vi "Panel.vi"(11 "SerialConfigPanel in":refnum<class "SerialConfigPanel.lvclass">) -> ()   [LabVIEW 2020, in "LV-Term.lvlib" / "SerialConfigPanel.lvclass"]
uses:
  SerialConfigPanel.lvclass
  SerialConfigPanel.lvclass/SerialConfigPanel.ctl
  <vilib>/IlluminatedG/IG OOPanel/OOPanel/Panel/Basic UI State.ctl
  <vilib>/IlluminatedG/IG OOPanel/OOPanel/Panel/Panel.lvclass
  <vilib>/IlluminatedG/IG OOPanel/OOPanel/OOPanel.lvlib
  C:/Program Files (x86)/National Instruments/LabVIEW 2020/vi.lib/IlluminatedG/IG OOPanel/OOPanel/Panel/Panel.lvclass
  C:/dev/illuminated-g/lv-terminal-app/LV-Term/SerialConfigPanel/SerialConfigPanel.lvclass
  C:/dev/illuminated-g/lv-terminal-app/LV-Term/ConfigPanel/ConfigPanel.lvclass
  <vilib>/IlluminatedG/IG Serial Stream/Stream-Serial/Serial Client/Stop Bits.ctl
  <vilib>/IlluminatedG/IG Serial Stream/Stream-Serial/Serial Client/Serial Client.lvclass
  <vilib>/IlluminatedG/IG Serial Stream/Stream-Serial/Serial Client/Flow Control.ctl
  <vilib>/IlluminatedG/IG Serial Stream/Stream-Serial/Serial Client/Parity.ctl
panel:
  in  "Port":refnum<visa-resource-name>
  in  "Timeout ms":i32=10000
  in  "Parity":T1
  in  "Flow Control":T2 items=["None", "XON/XOFF", "RTS/CTS", "XON/XOFF & RTS/CTS", "DTR/DSR", "XON/XOFF & DTR/DSR"]
  in  "Stop Bits":T3=10 items=["1.0"=10, "1.5"=15, "2.0"=20]
  in  "Data Bits":u8=8
  in  "Baud":u32=115200
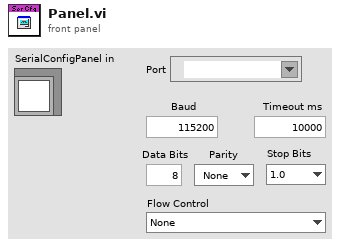
[diagram p1: front panel]
types:
  T1 = typedef "Stream-Serial.lvlib/Serial Client.lvclass/Parity.ctl" = enum16{"None", "Odd", "Even", "Mark", "Space"}
  T2 = typedef "Stream-Serial.lvlib/Serial Client.lvclass/Flow Control.ctl" = u16
  T3 = typedef "Stream-Serial.lvlib/Serial Client.lvclass/Stop Bits.ctl" = u16
  T4 = typedef "OOPanel.lvlib/Panel.lvclass/Basic UI State.ctl" = enum16{"Init", "Run", "Close"}
  T5 = typedef "OOPanel.lvlib/Panel.lvclass/Panel Events.ctl" = cluster{"Visbility":refnum<user-event>, "Close":refnum<user-event>}
  T6 = typedef "LV-Term.lvlib/SerialConfigPanel.lvclass/Ref Data.ctl" = cluster{"Port":refnum<visa-resource-name>, "Config":T7}
  T7 = typedef "Stream-Serial.lvlib/Serial Client.lvclass/Port Config.ctl" = cluster{"Baud (115200)":u32, "Data Bits (8)":u8, "Stop Bits (1)":T3, "Flow Control":T2, "Use LineTerm?":bool, "LineTerm (\\n)":string, "Timeout ms (10000)":i32, "Parity (None)":T1}
  T8 = typedef "OOPanel.lvlib/Panel.lvclass/Visibility State.ctl" = enum16{"Idle", "Closed", "Hidden", "Visible", "Subpanel"}
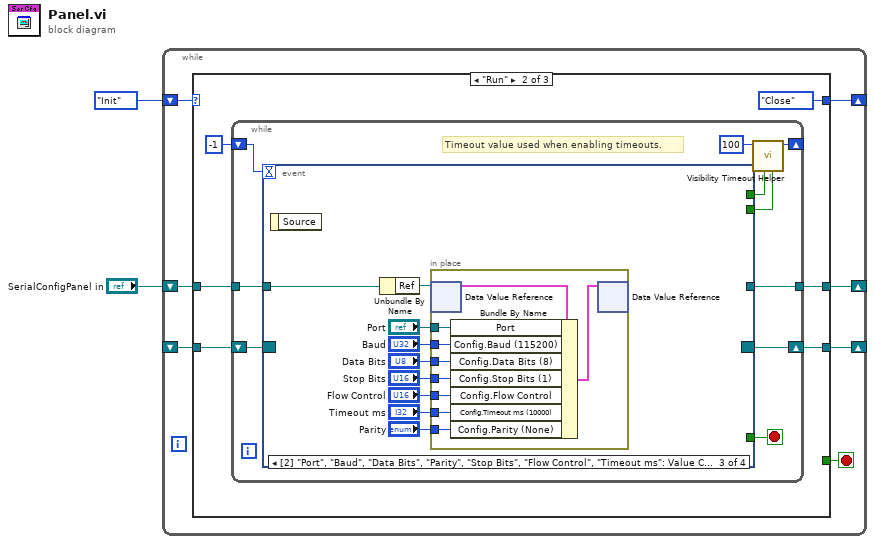
[diagram p0: block diagram]
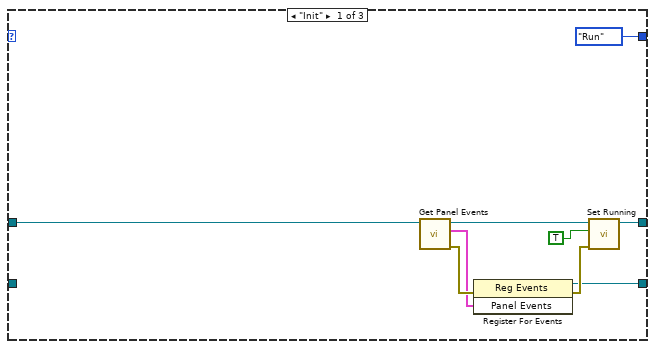
[diagram p2: hidden frame]
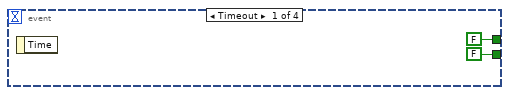
[diagram p3: hidden frame]
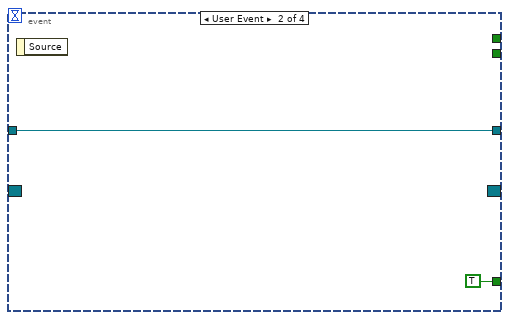
[diagram p4: hidden frame]
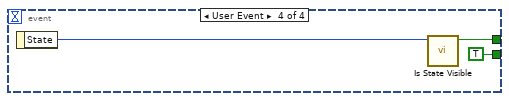
[diagram p5: hidden frame]
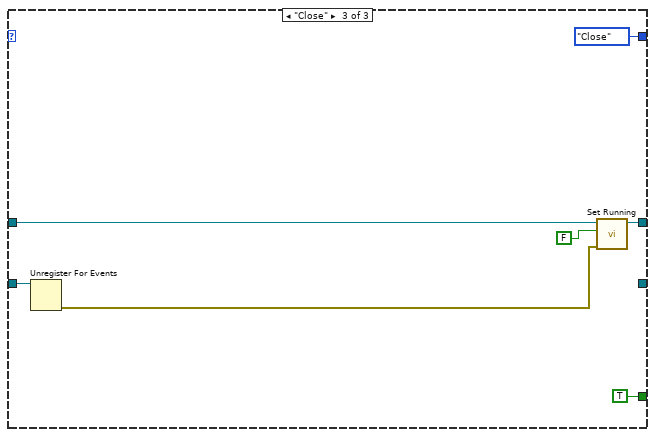
[diagram p6: hidden frame]
diagram:
  n1 = while {
    shift-right: [w8] -> _
    shift-left: _ -> [w9]
    shift-right: [w6] -> _
    shift-left: Basic_UI_State."Init" ("Basic UI State") -> [w7]
    shift-right: [w4] -> _
    shift-left: "SerialConfigPanel in" -> [w3]
    stop <- w5 stop-if-true
    n2 = case shown="\"Run\"" w7 {
      tunnel: w9 -> [_ w24 w62]
      tunnel: [w12 w22 _] -> w8
      tunnel: [Basic_UI_State."Run" ("Basic UI State") Basic_UI_State."Close" ("Basic UI State") Basic_UI_State."Close" ("Basic UI State")] -> w6
      tunnel: [_ _ TRUE] -> w5
      tunnel: [w11 w19 w60] -> w4
      tunnel: w3 -> [w10 w20 w61]
      frame "Init" {
        n3 = call <vilib>:"Get Panel Events.vi"("Panel in"=w10) -> ("error out"=w18:errorcluster, "Panel Events"=w14:T5, "Panel out"=w15:refnum<class "SerialConfigPanel.lvclass">)  [unwired: 8 in]
        n4 = register-events(error in=w18, w14) -> (reference out=w12:refnum<event-registration>, error out=w16:errorcluster)  [unwired: 1 in]
        n5 = call <vilib>:"Set Running.vi"("error in (no error)"=w16, "Running"=TRUE, "Panel in"=w15) -> ("Panel out"=w11:refnum<class "SerialConfigPanel.lvclass">)  [unwired: 7 in, 1 out]
      }
      frame "Run" {
        n6 = while {
          shift-right: [w30] -> w22
          shift-left: w24 -> [w31]
          shift-right: [w33] -> _
          shift-left: -1 ("Timeout") -> [w32]
          tunnel: w20 -> [w26]
          tunnel: [w25] -> w19
          stop <- w27 stop-if-true
          # "Timeout value used when enabling timeouts."
          n7 = event shown="[2] \"Port\", \"Baud\", \"Data Bits\", \"Parity\", \"Stop Bits\", \"Flow Control\", \"Timeout ms\": Value Change" {
            selector: w31 -> [_ _ _ _]
            dyn-events: [_ _ _ _] -> w30
            timeout: w32 -> [_ _ _ _]
            tunnel: [FALSE _ _ w58] -> w29
            tunnel: [FALSE _ _ TRUE] -> w28
            tunnel: [_ TRUE _ _] -> w27
            tunnel: w26 -> [_ w37 w46 _]
            tunnel: [_ w37 _ _] -> w25
            event Timeout {
              n8 = event-data() -> ()  [unwired: 1 in, 1 out]
            }
            event User Event {
              n9 = event-data() -> ()  [unwired: 1 in, 1 out]
            }
            event "Port", "Baud", "Data Bits", "Timeout ms": Value Change {
              n10 = event-data() -> ()  [unwired: 1 in, 1 out]
              n11 = Unbundle By Name(w46) -> ("Ref"=w47:refnum<data-value>)
              n12 = in-place {
                in-place-border: "Port" -> [w54]
                in-place-border: "Baud" -> [w53]
                in-place-border: "Data Bits" -> [w52]
                in-place-border: "Stop Bits" -> [w51]
                in-place-border: "Flow Control" -> [w50]
                in-place-border: "Timeout ms" -> [w49]
                in-place-border: "Parity" -> [w48]
                n13 = in-place-dvr #1(w47) -> (w56:T6)  [unwired: 1 out]
                n14 = Bundle By Name(cluster=w56, "Port"=w54, "Config.Baud (115200)"=w53, "Config.Data Bits (8)"=w52, "Config.Stop Bits (1)"=w51, "Config.Flow Control"=w50, "Config.Timeout ms (10000)"=w49, "Config.Parity (None)"=w48) -> (w55:T6)
                n15 = in-place-dvr #1(w55) -> ()  [unwired: 2 out]
              }
            }
            event User Event {
              n16 = event-data() -> ("State"=w59:T8)  [unwired: 1 in]
              n17 = call <vilib>:"Is State Visible.vi"("Visibility"=w59) -> ("Visible"=w58:bool)  [unwired: 10 in]
            }
          }
          n18 = call <vilib>:"Visibility Timeout Helper.vi"("Update?"=w28, "Use Timeout?"=w29, "Visible Timeout mS"=100) -> ("Timeout"=w33:i32)  [unwired: 8 in]
        }
      }
      frame "Close" {
        n19 = Unregister For Events(event registration refnum=w62) -> (error out=w64:errorcluster)  [unwired: 1 in]
        n20 = call <vilib>:"Set Running.vi"("error in (no error)"=w64, "Running"=FALSE, "Panel in"=w61) -> ("Panel out"=w60:refnum<class "SerialConfigPanel.lvclass">)  [unwired: 7 in, 1 out]
      }
    }
  }
